vi "Periodic Tasks.vi"(8 "error in":errorcluster) -> ()   [LabVIEW 2017]
doc: "This VI runs in parallel to other tasks. It can contain as many user-defined periodic loops as you need. These can carry out PID or other sorts of timed response."
uses:
  <vilib>/Rock Robotics/WPI/DriverStation/WPI_DriverStationRobotMode2.ctl
  <vilib>/Rock Robotics/WPI/Utilities/WPI_GetSetVariantRefNum.vi
  Robot Global Data.vi
  <vilib>/Rock Robotics/Network Tables/NT Write Number.vi
  <vilib>/Rock Robotics/WPI/ThirdParty/Phoenix-LabVIEW/Motor Controller/Get/CTRE_Phoenix_MotorController_GetPulseWidthAll.vi
  <vilib>/Rock Robotics/WPI/ThirdParty/Phoenix-LabVIEW/Motor Controller/Get/CTRE_Phoenix_MotorController_GetQuadratureData.vi
  <vilib>/Rock Robotics/Network Tables/NT Write Numeric Array.vi
  <vilib>/Rock Robotics/WPI/Solenoid/WPI_SolenoidGetEnum.vi
  <vilib>/Rock Robotics/WPI/RobotDrive/WPI_RobotDriveArcadeDrive_Standard(NoSaturation).vi
  navx-mxp/labview/navX Library v2/navX Library v2.lvlib
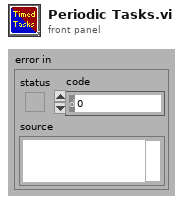
[diagram p1: front panel]
types:
  T1 = typedef "WPI_CompressorDevRef.ctl" = cluster{"DevStatus":errorcluster, "Pneumatics Control Module":u8}
  T2 = typedef "navX Library v2.lvlib/Z900_navX_DeviceTypeDef.ctl" = cluster{"Interface":cluster{"Protocol":T3, "Update Rate (4Hz-100Hz)":u8, "navX Open TypeDef":variant}, "Notify Packet":refnum<notifier>, "Loop VI Refnum":refnum<vi>, "Ready to Close Occurrence Refnum":refnum<k4>}
  T3 = typedef "navX Library v2.lvlib/Z900_navX_ProtocolTypeDef.ctl" = enum16{"SERIAL", "I2C", "SPI"}
  T4 = typedef "WPI_JoystickDevRef.ctl" = cluster{"Device":T5}
  T5 = typedef "WPI_JoystickDeviceEnum.ctl" = enum16{"USB 0", "USB 1", "USB 2", "USB 3", "USB 4", "USB 5"}
  T6 = typedef "WPI_MotorControlDeviceRef.ctl" = cluster{"DeviceStatus":errorcluster, "Type":T7, "PWM":cluster{"PWM Channel":T8, "DeadBand":T9}, "CAN":cluster{"Device Number":u8, "SetOutput VI Ref":variant, "GetOutput VI Ref":variant, "Enable VI Ref":variant, "Disable VI Ref":variant, "Data":variant}, "Invert":bool, "DIO PWM":cluster{"PWM \"Enable\" Channel":T8, "DIOChannel":T10, "PWM Rate":dbl}}
  T7 = typedef "WPI_MotorControlType.ctl" = enum16{"PWM", "CAN", "DIO PWM"}
  T8 = typedef "FPGA_DIOPWMChannel.ctl" = enum8{"PWM 0", "PWM 1", "PWM 2", "PWM 3", "PWM 4", "PWM 5", "PWM 6", "PWM 7", "PWM 8", "PWM 9", "PWM MXP 0", "PWM MXP 1", "PWM MXP 2", "PWM MXP 3", "PWM MXP 4", "PWM MXP 5", "PWM MXP 6", "PWM MXP 7", "PWM MXP 8", "PWM MXP 9", "Invalid"}
  T9 = typedef "WPI_PWMDeadband.ctl" = cluster{"Name":string, "maxPositivePwm":i32, "minPositivePwm":i32, "centerPwm":i32, "maxNegativePwm":i32, "minNegativePwm":i32, "angularRange":u16}
  T10 = typedef "FPGA_DIOChannel.ctl" = enum8{"DIO 0", "DIO 1", "DIO 2", "DIO 3", "DIO 4", "DIO 5", "DIO 6", "DIO 7", "DIO 8", "DIO 9", "DIO MXP 0", "DIO MXP 1", "DIO MXP 2", "DIO MXP 3", "DIO MXP 4", "DIO MXP 5", "DIO MXP 6", "DIO MXP 7", "DIO MXP 8", "DIO MXP 9", "DIO MXP 10", "DIO MXP 11", "DIO MXP 12", "DIO MXP 13", "DIO MXP 14", "DIO MXP 15", "SPI Port CS1", "SPI Port CS2", "SPI Port CS3", "SPI Port MISO", "SPI Port MOSI", "Invalid"}
  T11 = typedef "WPI_SolenoidDevRef.ctl" = cluster{"DevStatus":errorcluster, "Pneumatics Control Module":u8, "Forward Solenoid Channel":T12, "Reverse Solenoid Channel":T12}
  T12 = typedef "WPI_SolenoidChannel.ctl" = enum8{"Solenoid 0", "Solenoid 1", "Solenoid 2", "Solenoid 3", "Solenoid 4", "Solenoid 5", "Solenoid 6", "Solenoid 7", "Invalid"}
  T13 = typedef "WPI_RobotDriveDevRef.ctl" = cluster{"DevStatus":errorcluster, "Motors[]":T6[], "Square Inputs":bool, "Max Output":dbl}
  T14 = cluster{"navX Device":T2, "JoystickDevRef":T4, "RobotDriveDevRef":T13, "PhoenixMotorControlDevRef":T6, "PhoenixMotorControlDevRef":T6, "PhoenixMotorControlDevRef":T6, "PhoenixMotorControlDevRef":T6, "PhoenixMotorControlDevRef":T6, "PhoenixMotorControlDevRef":T6, "SolenoidDevRef":T11}
  T15 = typedef "WPI_DriverStationRobotMode2.ctl" = enum16{"Autonomous Disabled", "Autonomous Enabled", "Teleop Disabled", "Teleop Enabled", "Disconnected", "Finish", "Test Disabled", "Test Enabled", "Emergency Stopped"}
  T16 = cluster{"Yaw":dbl, "Roll":dbl, "Pitch":dbl, "Heading":dbl, "Fused Heading":dbl}
  T17 = typedef "WPI_GyroDevRef.ctl" = cluster{"DevStatus":errorcluster, "Analog Channel":T18, "Gain (VoltsPerDegree/Second)":dbl, "Gyro Type":enum16{"Analog", "XRS450"}, "Handle":i32, "SPI Bus":T19, "Device Found":bool, "Sample Rate":dbl, "Calibrate On Open":bool, "Offset":dbl}
  T18 = typedef "FPGA_AIChannel.ctl" = enum8{"AI 0", "AI 1", "AI 2", "AI 3", "AI MXP 0", "AI MXP 1", "AI MXP 2", "AI MXP 3", "Invalid"}
  T19 = typedef "spi_bus.ctl" = enum16{"SPI On-Board, CS0", "SPI On-Board, CS1", "SPI On-Board, CS2", "SPI On-Board, CS3", "SPI MXP", "Invalid"}
  T20 = typedef "WPI_SolenoidValue.ctl" = enum16{"Off", "On", "Forward", "Reverse"}
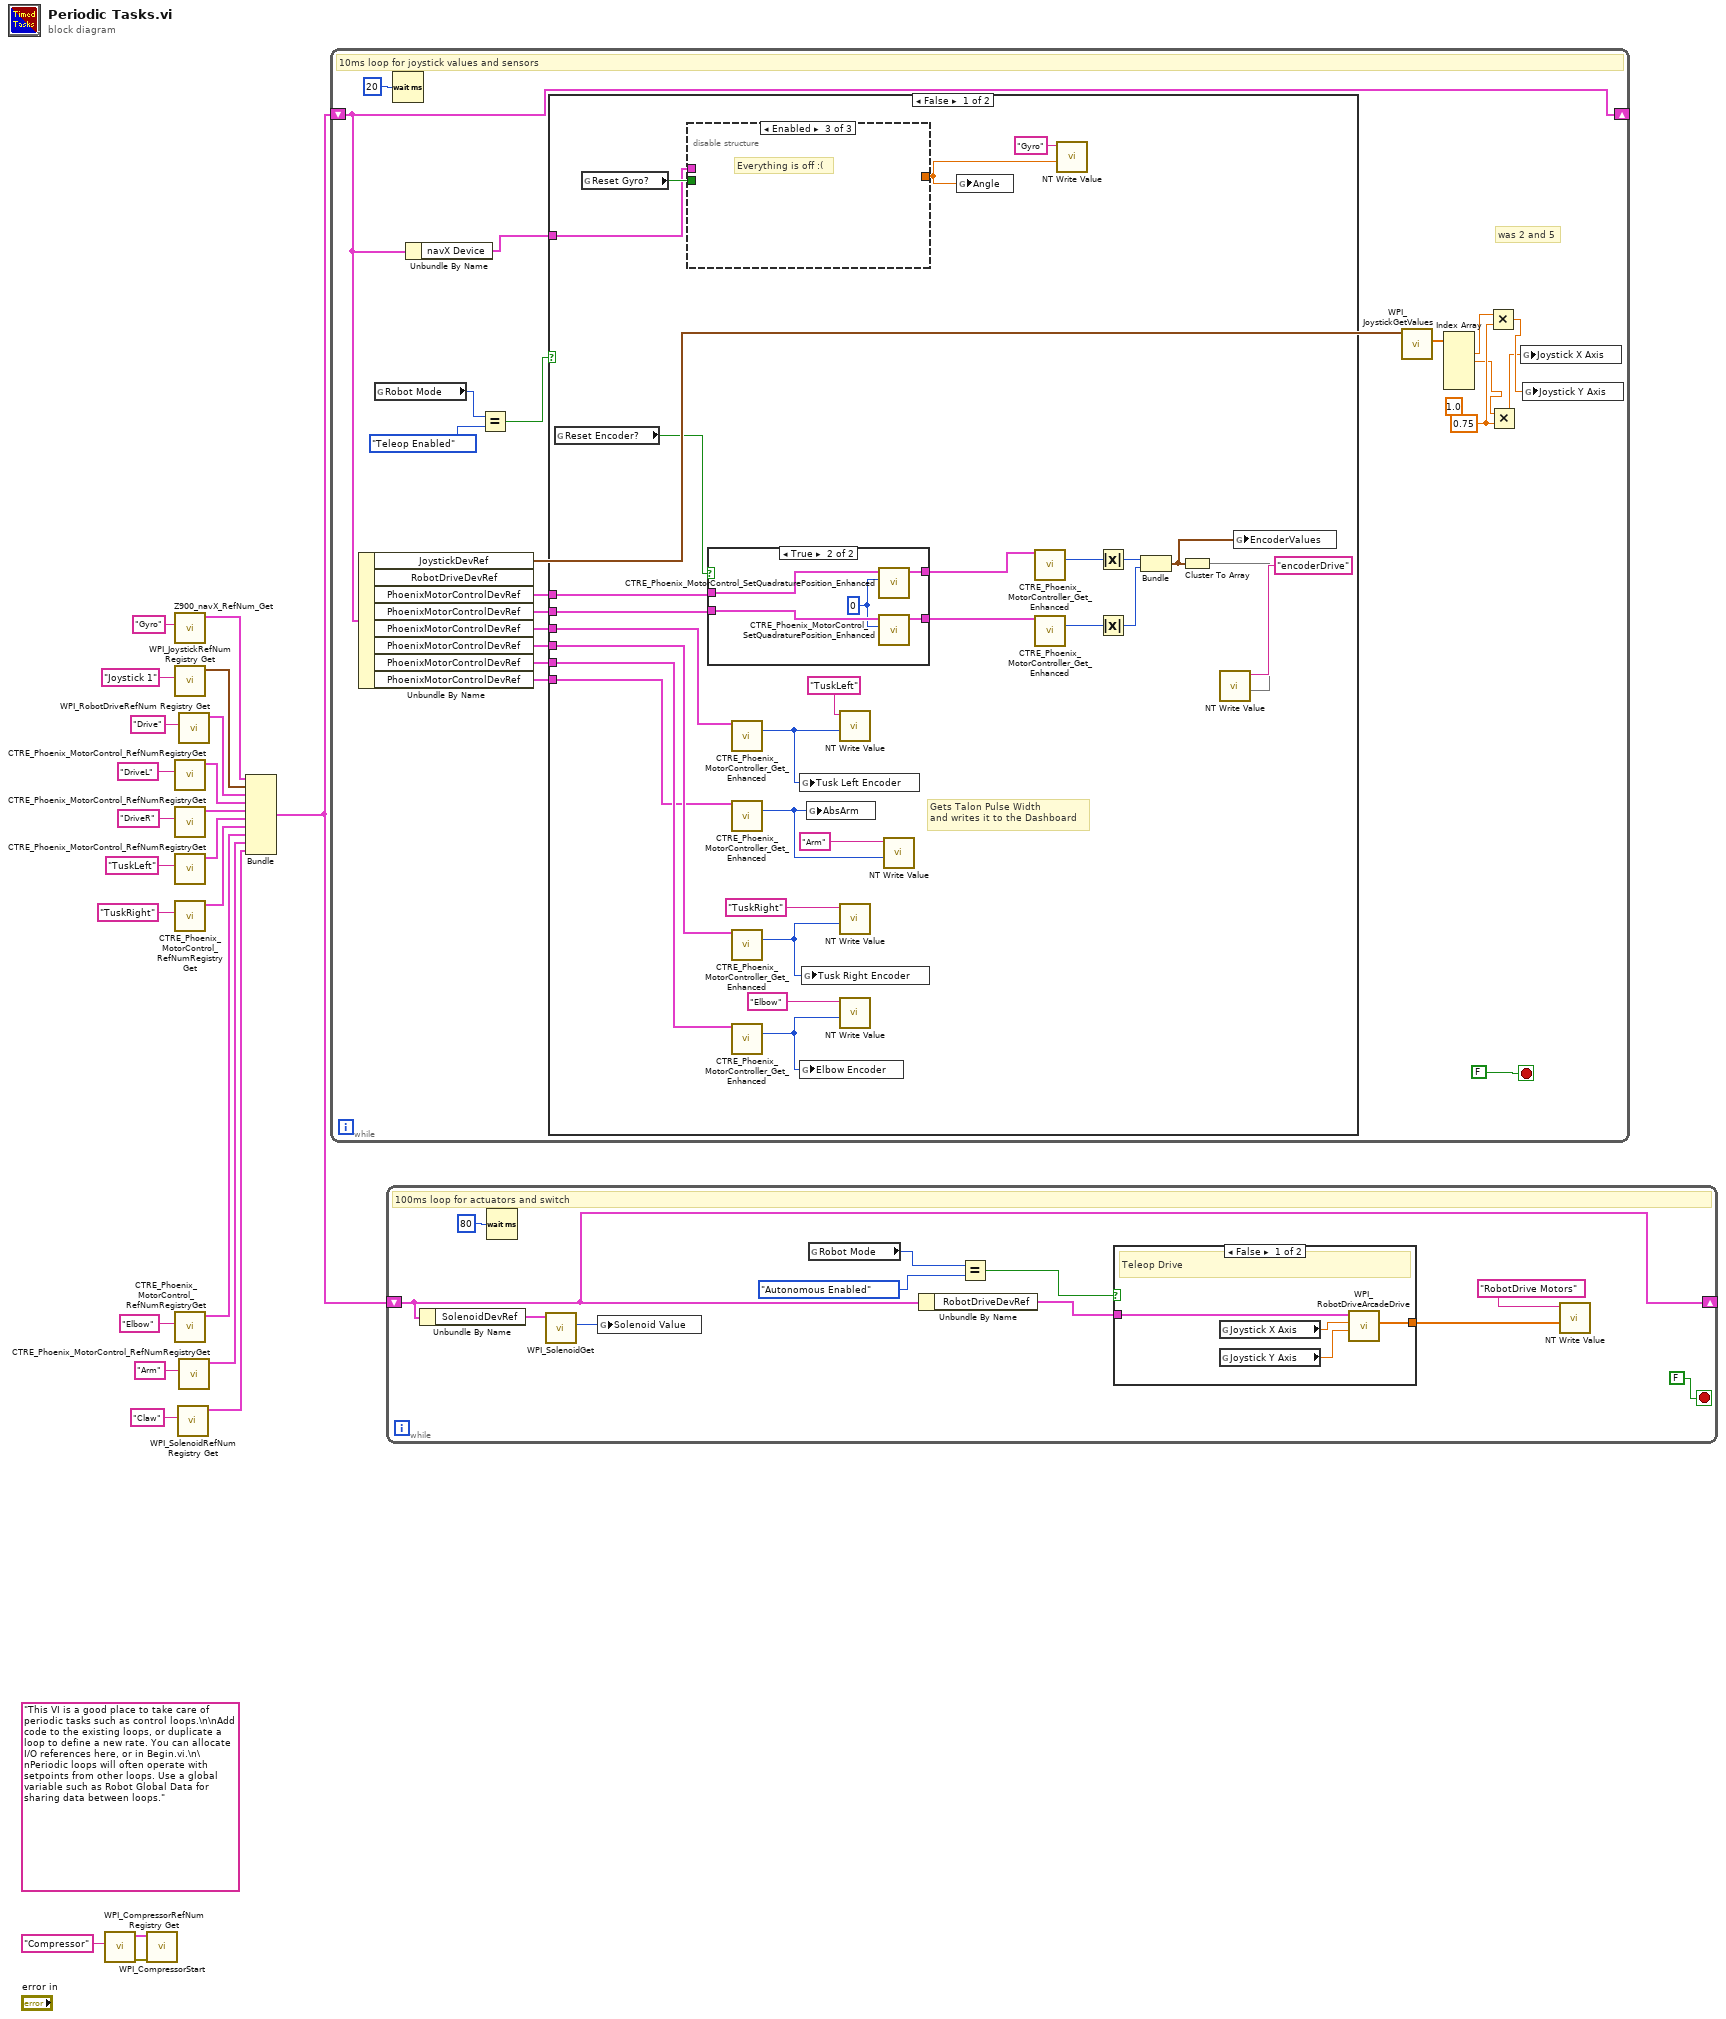
[diagram p0: block diagram]
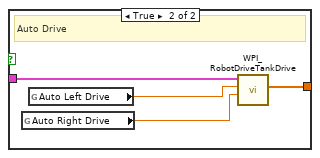
[diagram p2: hidden frame]
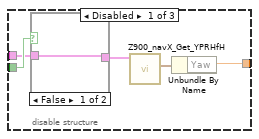
[diagram p3: hidden frame]
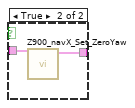
[diagram p4: hidden frame]
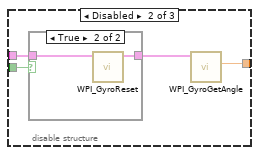
[diagram p5: hidden frame]
diagram:
  (unwired) "This VI is a good place to take care of periodic tasks such as control loops.\n\nAdd code to the existing loops, or duplicate a loop to define a new rate. You can allocate I/O references here, or in Begin.vi.\n\nPeriodic loops will often operate with setpoints from other loops. Use a global variable such as Robot Global Data for sharing data between loops."
  n1 = call <vilib>:"WPI_CompressorRefNum Registry Get.vi"("refnum name"="Compressor") -> ("error out"=w21:errorcluster, "CompressorDevRef"=w20:T1)  [unwired: 9 in]
  n2 = call <vilib>:"WPI_CompressorStart.vi"("error in (no error)"=w21, "CompressorDevRef"=w20) -> ()  [unwired: 8 in, 2 out]
  n3 = call "Z900_navX_RefNum_Get.vi"("refnum name"="Gyro") -> ("navX Device"=w1:T2)  [unwired: 9 in, 1 out]
  n4 = call <vilib>:"WPI_JoystickRefNum Registry Get.vi"("refnum name"="Joystick 1") -> ("JoystickDevRef"=w12:T4)  [unwired: 1 in, 9 out]
  n5 = call <vilib>:"CTRE_Phoenix_MotorControl_RefNumRegistryGet.vi"("refnum name"="DriveL") -> ("PhoenixMotorControlDevRef"=w10:T6)  [unwired: 9 in, 1 out]
  n6 = call <vilib>:"CTRE_Phoenix_MotorControl_RefNumRegistryGet.vi"("refnum name"="DriveR") -> ("PhoenixMotorControlDevRef"=w9:T6)  [unwired: 9 in, 1 out]
  n7 = call <vilib>:"CTRE_Phoenix_MotorControl_RefNumRegistryGet.vi"("refnum name"="TuskLeft") -> ("PhoenixMotorControlDevRef"=w8:T6)  [unwired: 9 in, 1 out]
  n8 = call <vilib>:"CTRE_Phoenix_MotorControl_RefNumRegistryGet.vi"("refnum name"="TuskRight") -> ("PhoenixMotorControlDevRef"=w7:T6)  [unwired: 9 in, 1 out]
  n9 = call <vilib>:"CTRE_Phoenix_MotorControl_RefNumRegistryGet.vi"("refnum name"="Elbow") -> ("PhoenixMotorControlDevRef"=w6:T6)  [unwired: 9 in, 1 out]
  n10 = call <vilib>:"WPI_SolenoidRefNum Registry Get.vi"("refnum name"="Claw") -> ("SolenoidDevRef"=w4:T11)  [unwired: 9 in, 1 out]
  n11 = call <vilib>:"WPI_RobotDriveRefNum Registry Get.vi"("refnum name"="Drive") -> ("RobotDriveDevRef"=w11:T13)  [unwired: 1 in, 9 out]
  n12 = call <vilib>:"CTRE_Phoenix_MotorControl_RefNumRegistryGet.vi"("refnum name"="Arm") -> ("PhoenixMotorControlDevRef"=w5:T6)  [unwired: 9 in, 1 out]
  n13 = Bundle("navX Device"=w1, "JoystickDevRef"=w12, "RobotDriveDevRef"=w11, "PhoenixMotorControlDevRef"=w10, "PhoenixMotorControlDevRef"=w9, "PhoenixMotorControlDevRef"=w8, "PhoenixMotorControlDevRef"=w7, "PhoenixMotorControlDevRef"=w6, "PhoenixMotorControlDevRef"=w5, "SolenoidDevRef"=w4) -> (w3:T14)  [unwired: 1 in]
  n14 = while {
    shift-right: [w34] -> _
    shift-left: w3 -> [w34]
    stop <- FALSE stop-if-true
    w29 = 0.75 ("y")
    (unwired) 1.0
    # "was 2 and 5"
    # "10ms loop for joystick values and sensors"
    n15 = Unbundle By Name(w34) -> ("JoystickDevRef"=w41:T4, "PhoenixMotorControlDevRef"=w40:T6, "PhoenixMotorControlDevRef"=w39:T6, "PhoenixMotorControlDevRef"=w38:T6, "PhoenixMotorControlDevRef"=w37:T6, "PhoenixMotorControlDevRef"=w36:T6, "PhoenixMotorControlDevRef"=w35:T6)  [unwired: 1 out]
    n16 = global read "Robot Global Data.vi" "Robot Mode"() -> (w33:T15)
    n17 = Wait (ms)(milliseconds to wait=u32 20) -> ()  [unwired: 1 out]
    n18 = Unbundle By Name(w34) -> ("navX Device"=w30:T2)
    n19 = Equal?(x=w33, y=WPI_DriverStationRobotMode2."Teleop Enabled") -> (x = y?=w32:bool)
    n20 = case shown="False" w32 {
      tunnel: w40 -> [w58 _]
      tunnel: w39 -> [w57 _]
      tunnel: w38 -> [w56 _]
      tunnel: w37 -> [w55 _]
      tunnel: w36 -> [w54 _]
      tunnel: w35 -> [w53 _]
      tunnel: w30 -> [w45 _]
      frame False {
        # "Gets Talon Pulse Width\nand writes it to the Dashboard"
        n21 = global read "Robot Global Data.vi" "Reset Encoder?"() -> (w70:bool)
        n22 = global read "Robot Global Data.vi" "Reset Gyro?"() -> (w48:bool)
        n23 = disable-structure shown="Enabled" {
          disable-tunnel: w48 -> [w76 w84 _]
          disable-tunnel: [w77 w81 _] -> w46
          disable-tunnel: w45 -> [w73 w83 _]
          frame Disabled {
            n24 = case shown="False" w76 {
              tunnel: [w78 w80] -> w75
              tunnel: w73 -> [w78 w79]
              frame False {
              }
              frame True {
                n25 = call "Z900_navX_Set_ZeroYaw.vi"("navX Device"=w79) -> ("navX Device"=w80:T2)  [unwired: 9 in, 1 out]
              }
            }
            n26 = call "Z900_navX_Get_YPRHfH.vi"("navX Device"=w75) -> ("YRPHfH"=w74:T16)  [unwired: 7 in, 3 out]
            n27 = Unbundle By Name(w74) -> ("Yaw"=w77:dbl)
          }
          frame Disabled {
            n28 = case shown="True" w84 {
              tunnel: w83 -> [w85 w87]
              tunnel: [w85 w86] -> w82
              frame False {
              }
              frame True {
                n29 = call <vilib>:"WPI_GyroReset.vi"("GyroDevRef"=w87) -> ("GyroDevRef"=w86:T17)  [unwired: 9 in, 1 out]
              }
            }
            n30 = call <vilib>:"WPI_GyroGetAngle.vi"("GyroDevRef"=w82) -> ("Angle"=w81:dbl)  [unwired: 6 in, 4 out]
          }
          frame Enabled {
            # "Everything is off :("
          }
        }
        n31 = case shown="True" w70 {
          tunnel: w58 -> [w89 w94]
          tunnel: w57 -> [w88 w92]
          tunnel: [w89 w93] -> w72
          tunnel: [w88 w91] -> w71
          frame False {
          }
          frame True {
            w90 = 0 ("New Position")
            n32 = call <vilib>:"CTRE_Phoenix_MotorControl_SetQuadraturePosition_Enhanced.vi"("New Position"=w90, "PhoenixMotorControlDevRef"=w94) -> ("PhoenixMotorControlDevRef"=w93:T6)  [unwired: 8 in, 1 out]
            n33 = call <vilib>:"CTRE_Phoenix_MotorControl_SetQuadraturePosition_Enhanced.vi"("New Position"=w90, "PhoenixMotorControlDevRef"=w92) -> ("PhoenixMotorControlDevRef"=w91:T6)  [unwired: 8 in, 1 out]
          }
        }
        n34 = call-poly <vilib>:"CTRE_Phoenix_MotorController_Get_Enhanced.vi"("PhoenixMotorControlDevRef"=w56) -> ("Pulse Width Position"=w49:i32)  [unwired: 9 in, 5 out]
        n35 = call-poly <vilib>:"CTRE_Phoenix_MotorController_Get_Enhanced.vi"("PhoenixMotorControlDevRef"=w53) -> ("Pulse Width Position"=w52:i32)  [unwired: 9 in, 5 out]
        n36 = call-poly <vilib>:"CTRE_Phoenix_MotorController_Get_Enhanced.vi"("PhoenixMotorControlDevRef"=w55) -> ("Pulse Width Position"=w50:i32)  [unwired: 9 in, 5 out]
        n37 = call-poly <vilib>:"CTRE_Phoenix_MotorController_Get_Enhanced.vi"("PhoenixMotorControlDevRef"=w54) -> ("Pulse Width Position"=w51:i32)  [unwired: 9 in, 5 out]
        n38 = global write "Robot Global Data.vi" "Tusk Left Encoder"(w49) -> ()
        n39 = global write "Robot Global Data.vi" "Elbow Encoder"(w51) -> ()
        n40 = global write "Robot Global Data.vi" "Tusk Right Encoder"(w50) -> ()
        n41 = global write "Robot Global Data.vi" "AbsArm"(w52) -> ()
        n42 = call-poly <vilib>:"NT Write Value.vi"("Numeric"=w49, "Name"="TuskLeft") -> ()  [unwired: 9 in, 1 out]
        n43 = call-poly <vilib>:"NT Write Value.vi"("Numeric"=w50, "Name"="TuskRight") -> ()  [unwired: 9 in, 1 out]
        n44 = call-poly <vilib>:"NT Write Value.vi"("Numeric"=w51, "Name"="Elbow") -> ()  [unwired: 9 in, 1 out]
        n45 = call-poly <vilib>:"NT Write Value.vi"("Numeric"=w52, "Name"="Arm") -> ()  [unwired: 9 in, 1 out]
        n46 = global write "Robot Global Data.vi" "Angle"(w46) -> ()
        n47 = call-poly <vilib>:"CTRE_Phoenix_MotorController_Get_Enhanced.vi"("PhoenixMotorControlDevRef"=w72) -> ("Quadrature Position"=w66:i32)  [unwired: 11 in, 3 out]
        n48 = call-poly <vilib>:"CTRE_Phoenix_MotorController_Get_Enhanced.vi"("PhoenixMotorControlDevRef"=w71) -> ("Quadrature Position"=w69:i32)  [unwired: 11 in, 3 out]
        n49 = call-poly <vilib>:"NT Write Value.vi"("Numeric"=w46, "Name"="Gyro") -> ()  [unwired: 9 in, 1 out]
        n50 = Absolute Value(x=w66) -> (abs(x)=w67:i32)
        n51 = Absolute Value(x=w69) -> (abs(x)=w68:i32)
        n52 = Bundle(w67, w68) -> (w60:cluster{i32, i32})  [unwired: 1 in]
        n53 = Cluster To Array(cluster=w60) -> (array=w59:i32[])
        n54 = call-poly <vilib>:"NT Write Value.vi"("Numeric Array"=w59, "Name"="encoderDrive") -> ()  [unwired: 9 in, 1 out]
        n55 = global write "Robot Global Data.vi" "EncoderValues"(w60) -> ()
      }
      frame True {
      }
    }
    n56 = call <vilib>:"WPI_JoystickGetValues.vi"("JoystickDevRef"=w41) -> ("Axes"=w42:dbl[])  [unwired: 6 in, 4 out]
    n57 = Index Array(array=w42) -> (element #1=w28:dbl, element #2=w27:dbl)  [unwired: 5 in, 3 out]
    n58 = Multiply(x=w28, y=w29) -> (x*y=w26:dbl)
    n59 = Multiply(x=w27, y=w29) -> (x*y=w25:dbl)
    n60 = global write "Robot Global Data.vi" "Joystick X Axis"(w25) -> ()
    n61 = global write "Robot Global Data.vi" "Joystick Y Axis"(w26) -> ()
  }
  n62 = while {
    shift-right: [w95] -> _
    shift-left: w3 -> [w95]
    stop <- FALSE stop-if-true
    # "100ms loop for actuators and switch"
    n63 = Unbundle By Name(w95) -> ("SolenoidDevRef"=w97:T11)
    n64 = Wait (ms)(milliseconds to wait=u32 80) -> ()  [unwired: 1 out]
    n65 = call-poly <vilib>:"WPI_SolenoidGet.vi"("SolenoidDevRef"=w97) -> ("Value"=w96:T20)  [unwired: 8 in, 2 out]
    n66 = global write "Robot Global Data.vi" "Solenoid Value"(w96) -> ()
    n67 = global read "Robot Global Data.vi" "Robot Mode"() -> (w102:T15)
    n68 = Unbundle By Name(w95) -> ("RobotDriveDevRef"=w100:T13)
    n69 = Equal?(x=w102, y=WPI_DriverStationRobotMode2."Autonomous Enabled") -> (x = y?=w103:bool)
    n70 = case shown="False" w103 {
      tunnel: w100 -> [w109 w110]
      tunnel: [w106 w113] -> w98
      frame False {
        # "Teleop Drive"
        n71 = global read "Robot Global Data.vi" "Joystick X Axis"() -> (w108:dbl)
        n72 = global read "Robot Global Data.vi" "Joystick Y Axis"() -> (w107:dbl)
        n73 = call-poly <vilib>:"WPI_RobotDriveArcadeDrive.vi"("Y axis value"=w107, "X axis value"=w108, "RobotDriveDevRef"=w109) -> ("Motor Values"=w106:dbl[])  [unwired: 6 in, 2 out]
      }
      frame True {
        # "Auto Drive"
        n74 = global read "Robot Global Data.vi" "Auto Right Drive"() -> (w111:dbl)
        n75 = global read "Robot Global Data.vi" "Auto Left Drive"() -> (w112:dbl)
        n76 = call <vilib>:"WPI_RobotDriveTankDrive.vi"("Right axis value"=w111, "Left axis value"=w112, "RobotDriveDevRef"=w110) -> ("Motor Values"=w113:dbl[])  [unwired: 6 in, 2 out]
      }
    }
    n77 = call-poly <vilib>:"NT Write Value.vi"("Numeric Array"=w98, "Name"="RobotDrive Motors") -> ()  [unwired: 9 in, 1 out]
  }
